vi "Copy Pixmap to Image (ARGB Flatten Mask).vi"(7 "Colour (Default: Black)":T1={"Alpha"=255, "RGB"=0}, 8 "error in (no error)":errorcluster, 10 "ARGB Image Destination":T3, 11 "Pixmap Image Data":T2) -> (0 "error out":errorcluster, 3 "ARGB Image Destination (duplicate)":T3)   [LabVIEW 2020, in "g_ar_toolkit.image.lvlib"]
uses:
  g_ar_toolkit.image.lvlib
  ARGB Image.ctl
  <vilib>/picture/picture.llb/imagedata.ctl
  ARGB Colour.ctl
  7d03ccf7-b889-4e8d-9f2a-57831e73dbde.vi
  FixPixmap.vi
  Default8bitColourMap.vi
  <vilib>/Utility/error.llb/Error Cluster From Error Code.vi
  g_ar_toolkit.common/Module Path.vi
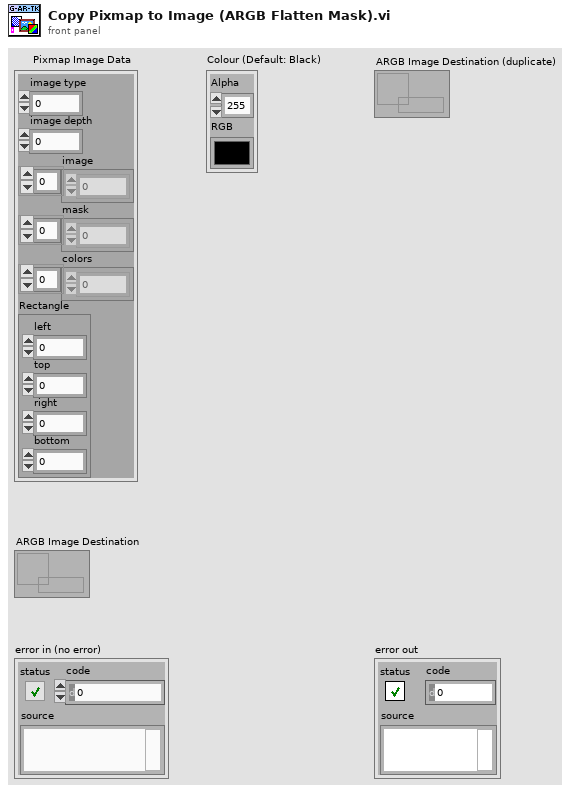
[diagram p1: front panel]
types:
  T1 = typedef "g_ar_toolkit.image.lvlib/ARGB Colour.ctl" = cluster{"Alpha":u8, "RGB":u32}
  T2 = typedef "imagedata.ctl" = cluster{"image type":i32, "image depth":i32, "image":u8[], "mask":u8[], "colors":u32[], "Rectangle":cluster{"left":i16, "top":i16, "right":i16, "bottom":i16}}
  T3 = typedef "g_ar_toolkit.image.lvlib/ARGB Image.ctl" = refnum<data-value>
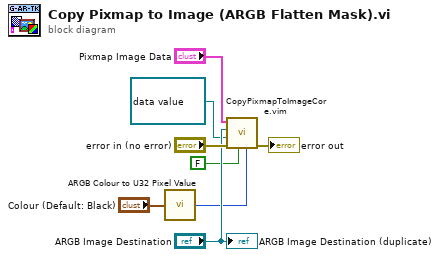
[diagram p0: block diagram]
diagram:
  n1 = call "ARGB Colour to U32 Pixel Value.vi"("ARGB Colour"="Colour (Default: Black)") -> ("U32 Colour"=w1:u32)
  n2 = call "CopyPixmapToImageCore.vim"("Background Value"=w1, "Has Mask"=FALSE, "error in (no error)"="error in (no error)", "Mask Image"=refnum<data-value> refnum ("ARGB Image Mask"), "Source Image"="ARGB Image Destination", "image data"="Pixmap Image Data") -> ("error out"=→"error out":errorcluster)  [unwired: 5 in]
  "ARGB Image Destination (duplicate)" <- "ARGB Image Destination"
